vi "Data.vi"(11 "Create Msg in":refnum<class "Create Msg.lvclass">) -> (1 "Alias":string, 2 "Actor":refnum<class "Actor.lvclass">)   [LabVIEW 2021, in "Create.lvlib" / "Create Msg.lvclass"]
uses:
  Create Msg.lvclass
  jettl/Actor/Actor.lvclass
  Create Msg.lvclass/Create Msg.ctl
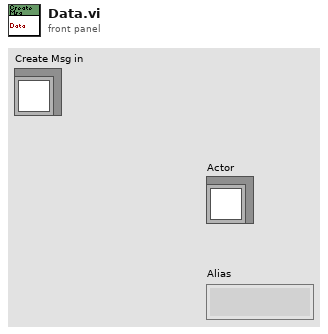
[diagram p1: front panel]
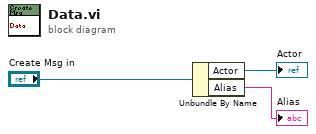
[diagram p0: block diagram]
diagram:
  n1 = Unbundle By Name("Create Msg in") -> ("Actor"=→"Actor":refnum<class "Actor.lvclass">, "Alias"=→"Alias":string)
